vi "test_Read I32 Register Value.vi"(8 "error in (no error)":errorcluster, 11 "TestCase in":refnum<class "FPGA Register IO Tests.lvclass">) -> (0 "error out":errorcluster, 3 "TestCase out":refnum<class "FPGA Register IO Tests.lvclass">)   [LabVIEW 2021, in "FPGA Register IO Tests.lvclass"]
uses:
  FPGA Register IO Tests.lvclass
  FPGA Register IO Tests.lvclass/FPGA Register IO Tests.ctl
  APIs/FPGA Register IO/Read Methods/Read Data Register/Instances/Read I32.vi
  APIs/FPGA Register IO/Utilities/Find Register Offset.vi
  APIs/FPGA Register IO/SubVIs/Check Register Data Store.vi
  APIs/FPGA Register IO/Error Handling/Error 6001.vi
  APIs/FPGA Register IO/Error Handling/Error 6000.vi
  APIs/FPGA Register IO/Error Handling/Error 6002.vi
  APIs/FPGA Register IO/Error Handling/Error 6003.vi
  <vilib>/FPGAPlugInAG/Dynamic/niLvFpga_Close_Dynamic.vi
  <vilib>/rvi/interface/nirviCloseFPGA/nirviCloseFPGA.xnode
  <vilib>/addons/_JKI Toolkits/VI Tester/TestCase.llb/TestCase.lvclass
  APIs/FPGA Register IO/FPGA Register IO.lvlib
  C:/Program Files/National Instruments/LabVIEW 2021/vi.lib/addons/_JKI Toolkits/VI Tester/TestCase.llb/TestCase.lvclass
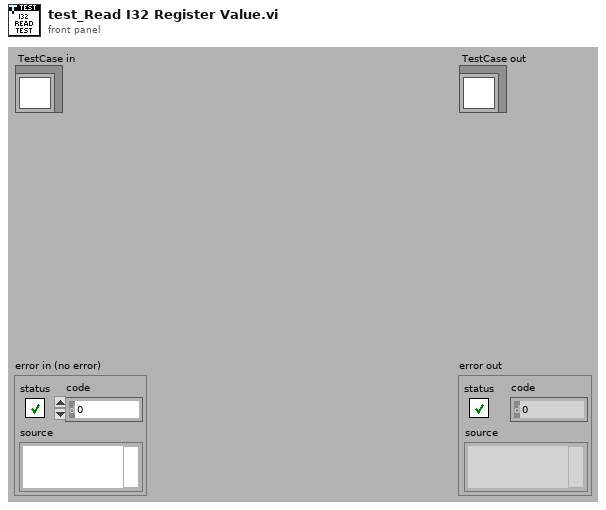
[diagram p1: front panel]
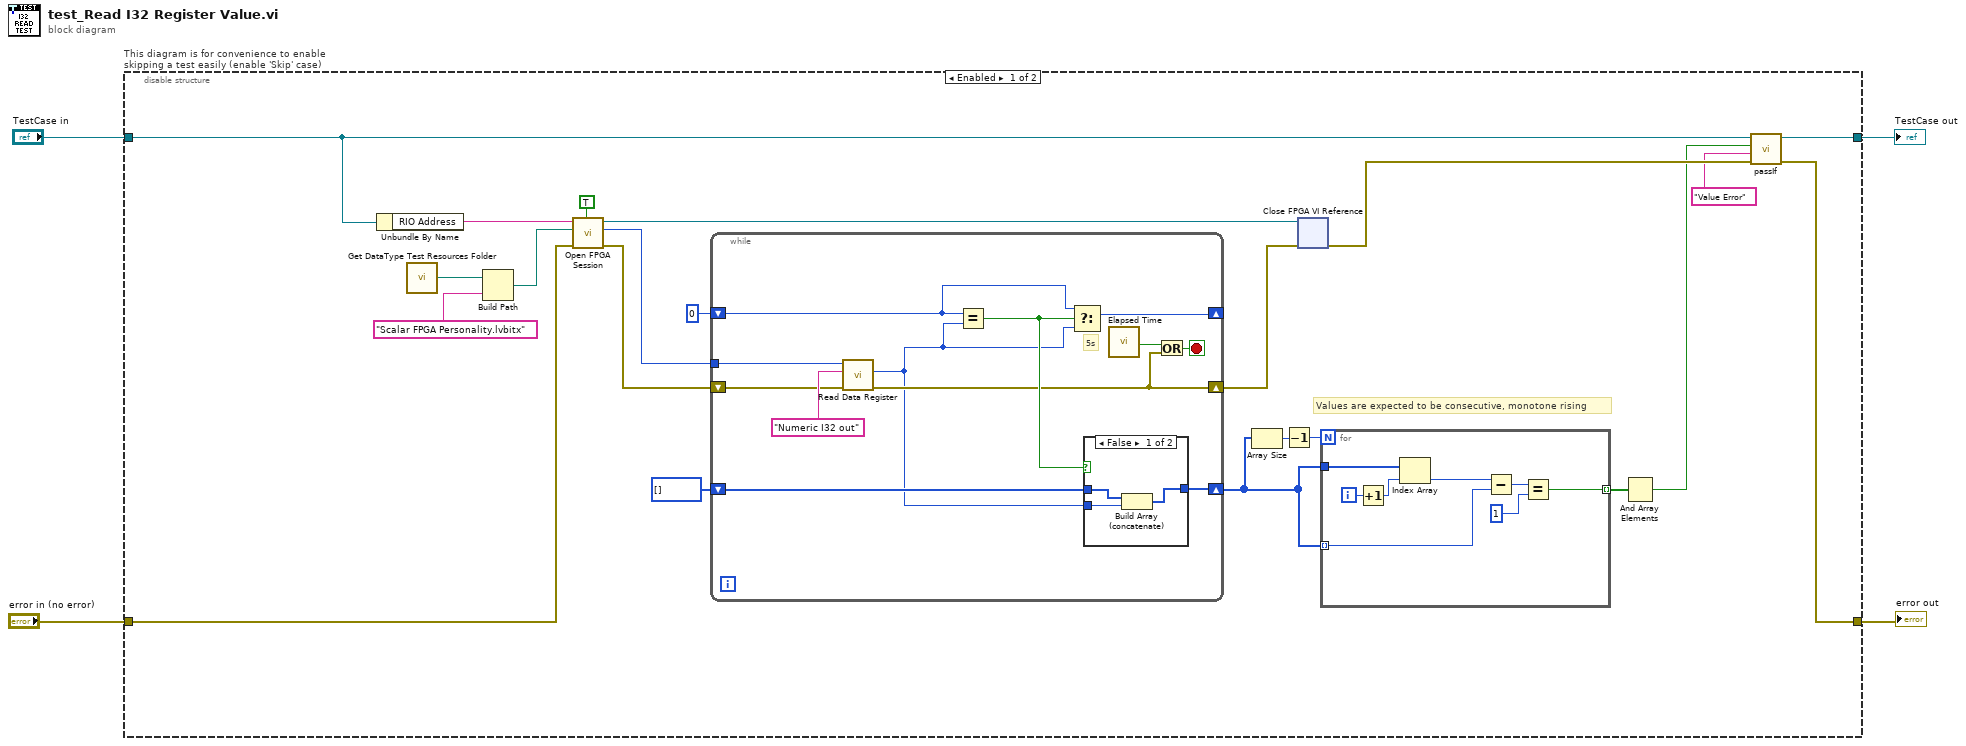
[diagram p0: block diagram]
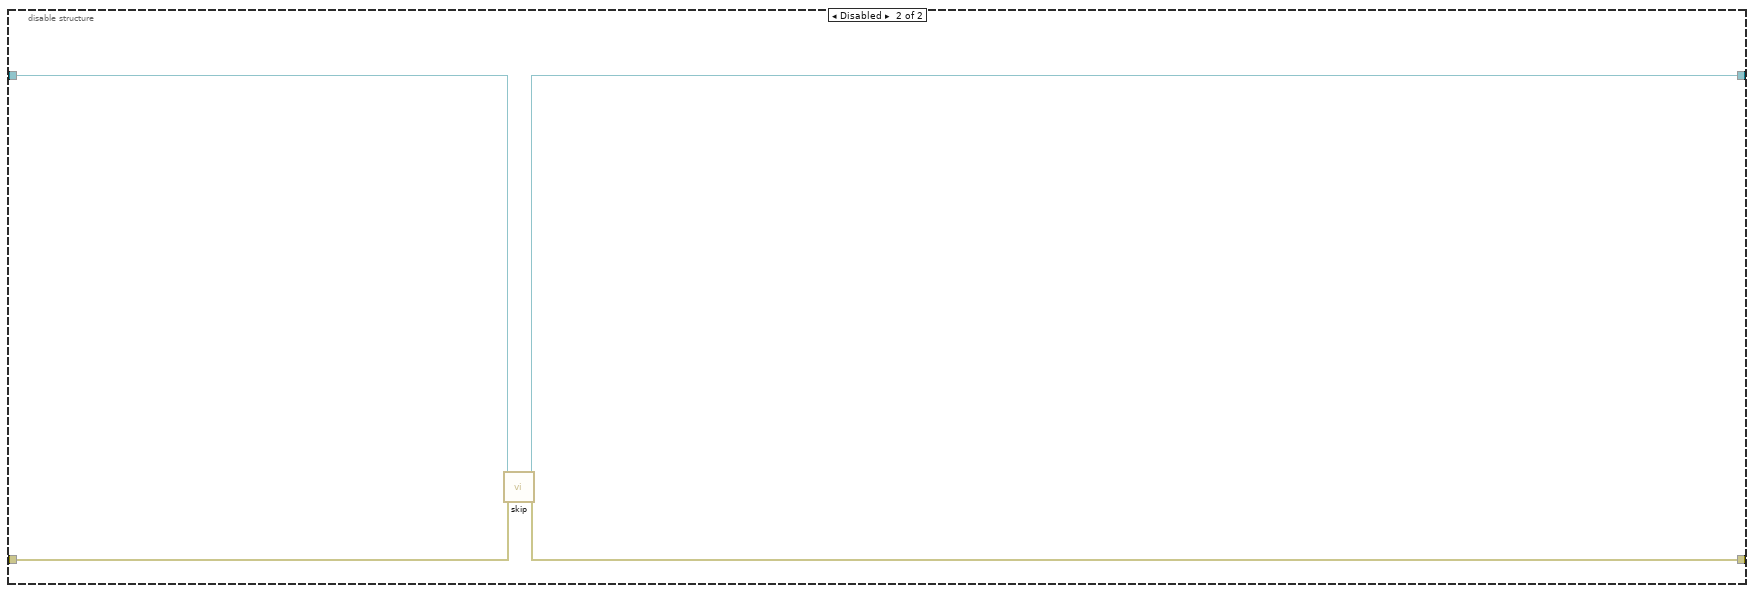
[diagram p3: hidden frame]
diagram:
  n1 = disable-structure "This diagram is for convenience to enable skipping a test easily (enable 'Skip' case)" shown="Enabled" {
    disable-tunnel: "TestCase in" -> [w12 w54]
    disable-tunnel: [w6 w52] -> w1
    disable-tunnel: [w5 w53] -> w3
    disable-tunnel: "error in (no error)" -> [w13 w51]
    frame Enabled {
      # "Values are expected to be consecutive, monotone rising"
      n2 = Unbundle By Name(w12) -> ("RIO Address"=w15:string)
      n3 = call "Get DataType Test Resources Folder.vi"() -> ("path"=w10:path)
      n4 = Build Path(base path=w10, name or relative path="Scalar FPGA Personality.lvbitx") -> (appended path=w14:path)
      n5 = call "Open FPGA Session.vi"("run when loaded (T)"=TRUE ("Run When Loaded (T)"), "error in"=w13, "bitfile path"=w14, "device address"=w15) -> ("error out"=w21:errorcluster, "session out"=w20:u32, "bitfile reference out"=w19:refnum<k20>)  [unwired: 5 in]
      n6 = while {
        tunnel: w20 -> [w33]
        shift-right: [w28] -> w18
        shift-left: w21 -> [w31]
        shift-right: [w37] -> _
        shift-left: 0 ("DBL Value") -> [w38]
        shift-right: [w35] -> w22
        shift-left: i32[] [] -> [w34]
        stop <- w30 stop-if-true
        # "5s"
        n7 = call-poly "Read Data Register.vi"("error in"=w31, "register name"="Numeric I32 out" ("registerName"), "session in"=w33) -> ("error out"=w28:errorcluster, "value out"=w27:i32)  [unwired: 6 in, 1 out]
        n8 = Equal?(x=w38, y=w27) -> (x = y?=w36:bool)
        n9 = Select(t=w38, s=w36, f=w27) -> (s? t:f=w37:i32)
        n10 = case shown="False" w36 {
          tunnel: w27 -> [w41 _]
          tunnel: [w40 w42] -> w35
          tunnel: w34 -> [w39 w42]
          frame False {
            n11 = Build Array (concatenate)(w39, w41) -> (w40:i32[])
          }
          frame True {
          }
        }
        n12 = call "Elapsed Time"() -> ("Time has Elapsed"=w29:bool)  [unwired: 12 in, 7 out]
        n13 = Or(x=w29, y=w28) -> (x .or. y?=w30:bool)
      }
      n14 = Array Size(array=w22) -> (size(s)=w23:i32)
      n15 = Decrement(x=w23) -> (x-1=w24:i32)
      n16 = xnode "Close FPGA VI Reference"("FPGA VI Reference In"=w19, "error in"=w18) -> ("error out"=w11:errorcluster)
      n17 = for {
        N: w24 -> [_]
        tunnel: w22 -> [w43] mode=indexing
        tunnel: w22 -> [w50]
        tunnel: [w45] -> w25 mode=indexing
        i -> [w49]
        n18 = Increment(x=w49) -> (x+1=w48:i32)
        n19 = Index Array(array=w50, index=w48) -> (element=w44:i32)
        n20 = Subtract(x=w44, y=w43) -> (x-y=w47:i32)
        n21 = Equal?(x=w47, y=1) -> (x = y?=w45:bool)
      }
      n22 = And Array Elements(Boolean array=w25) -> (logical AND=w9:bool)
      n23 = call-dynamic "passIf.vi"("error in (no error)"=w11, "message (\"\")"="Value Error" ("message (\"\")"), "pass"=w9, "TestCase in"=w12) -> ("error out"=w5:errorcluster, "TestCase out"=w6:refnum<class "FPGA Register IO Tests.lvclass">)  [unwired: 6 in]
    }
    frame Disabled {
      # "skip test result while test is under development"
      n24 = call <vilib>:"skip.vi"("error in (no error)"=w51, "TestCase in"=w54) -> ("error out"=w53:errorcluster, "TestCase out"=w52:refnum<class "FPGA Register IO Tests.lvclass">)  [unwired: 8 in]
    }
  }
  "error out" <- w3
  "TestCase out" <- w1
